vi "Set Sensor COM Port.vi"(8 "error in (no error)":errorcluster, 10 "COM Port":refnum<visa-resource-name>, 11 "Sensor in":refnum<class "Sensor.lvclass">) -> (0 "error out":errorcluster, 3 "Sensor out":refnum<class "Sensor.lvclass">)   [LabVIEW 2016, in "Sensor.lvlib" / "Sensor.lvclass"]
uses:
  Sensor.lvclass
  Sensor.lvclass/Sensor.ctl
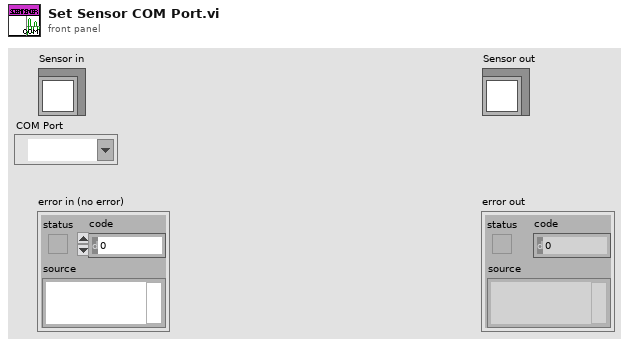
[diagram p1: front panel]
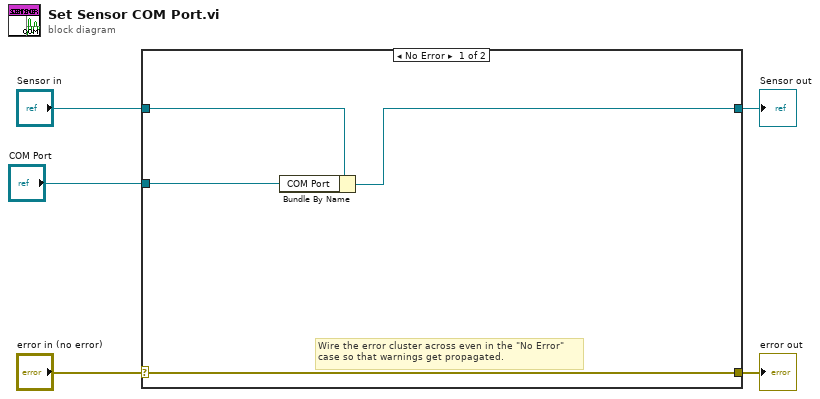
[diagram p0: block diagram]
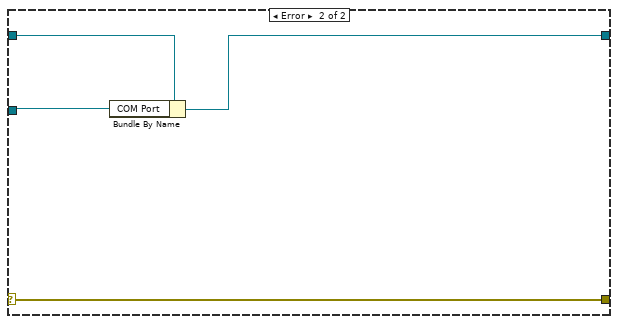
[diagram p2: hidden frame]
diagram:
  n1 = case shown="No Error" "error in (no error)" {
    selector: "error in (no error)" -> [w9 w13]
    tunnel: [w9 w13] -> w4
    tunnel: [w6 w10] -> w2
    tunnel: "Sensor in" -> [w8 w11]
    tunnel: "COM Port" -> [w7 w12]
    frame No Error {
      # "Wire the error cluster across even in the \"No Error\"\ncase so that warnings get propagated."
      n2 = Bundle By Name(cluster=w8, "COM Port"=w7) -> (w6:refnum<class "Sensor.lvclass">)
    }
    frame Error {
      n3 = Bundle By Name(cluster=w11, "COM Port"=w12) -> (w10:refnum<class "Sensor.lvclass">)
    }
  }
  "error out" <- w4
  "Sensor out" <- w2
